vi "RT target - PWM Example.vi"() -> ()   [LabVIEW 2013]
uses:
  <vilib>/Platform/TimedLoop/XDataNode/timing_clust.ctl
  <vilib>/Platform/TimedLoop/XDataNode/nitl_modes.ctl
  <vilib>/Platform/TimedLoop/XDataNode/wakeup.ctl
  <vilib>/FPGAPlugInAG/cRIO-9068/niLvFpga_Open_cRIO-9068.vi
  <vilib>/Utility/error.llb/Error Cluster From Error Code.vi
  <vilib>/rvi/errors/niLvFpgaAdjustHostInterfaceError.vi
  <vilib>/FPGAPlugInAG/cRIO-9068/niLvFpga_Close_cRIO-9068.vi
  <vilib>/platform/TimedLoop/XDataNode/XDataNode.xnode
  <vilib>/rvi/interface/nirviOpenFPGA/nirviOpenFPGA.xnode
  FPGA Bitfiles/testscanmode_FPGATarget_FPGA-PWMExample_nwIUPoe6BIw.lvbitx
  FPGA - PWM Example.vi
  <vilib>/rvi/interface/nirviReadWriteControl/nirviReadWriteControl.xnode
  <vilib>/rvi/interface/nirviCloseFPGA/nirviCloseFPGA.xnode
  <vilib>/Platform/TimedLoop/XDataNode/XDNodeRunTimeDep.lvlib
  NiFpgaLv.dll
panel:
  in  "Array":bool[](array[boolean])
  out "error out":errorcluster
  in  "stop":bool
  # "Pulse Width Modulation (PWM)\nNI 9474 (Slot 4)"
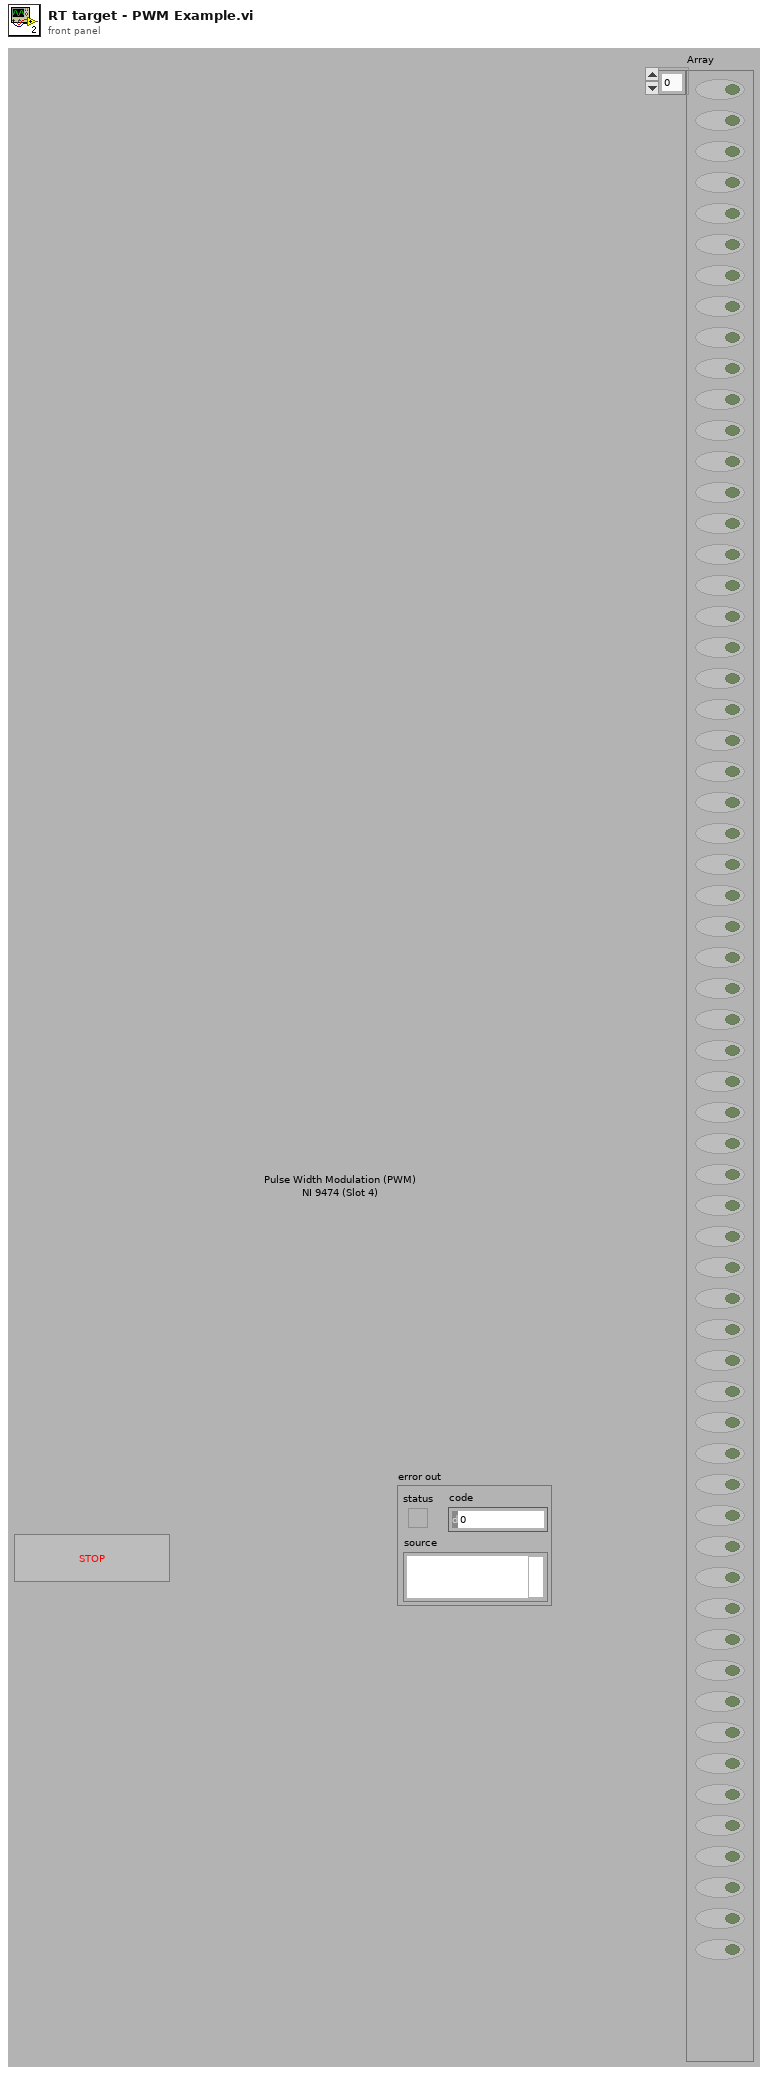
[diagram p1: front panel]
types:
  T1 = typedef "XDNodeRunTimeDep.lvlib/timing_clust.ctl" = cluster{"Expected End [f-1]":u64, "Actual End [f-1]":u64, "Finished Late? [f-1]":bool, "Expected End [i-1]":u64, "Actual End [i-1]":u64, "Finished Late? [i-1]":bool, "Expected Start [i]":u64, "Actual Start [i]":u64, "Expected Start [f]":u64, "Actual Start [f]":u64, "Source Name":string, "Structure Name":string, "Period":i64, "Deadline":i64, "Offset":i64, "Start":i64, "Priority":i32, "Timeout":i32, "Mode":T2, "Wakeup Reason":T3, "Error":errorcluster, "Source Type":string, "Secondary Source Type":string, "Global End Time":u64, "Global Start Time":u64, "Frame Duration":u64, "Iteration Duration":u64, "Assigned CPU":i32, "I/O Scan Engine Mode":u32}
  T2 = typedef "XDNodeRunTimeDep.lvlib/nitl_modes.ctl" = enum32{"No Change", "Process missed periods, maintain original phase", "Discard missed periods, maintain original phase", "Process missed periods, ignore original phase", "Discard missed periods, ignore original phase"}
  T3 = typedef "XDNodeRunTimeDep.lvlib/wakeup.ctl" = enum32{"Normal", "Aborted", "Asynchronous wakeup", "Timing source error", "Timed loop error", "Timeout"}
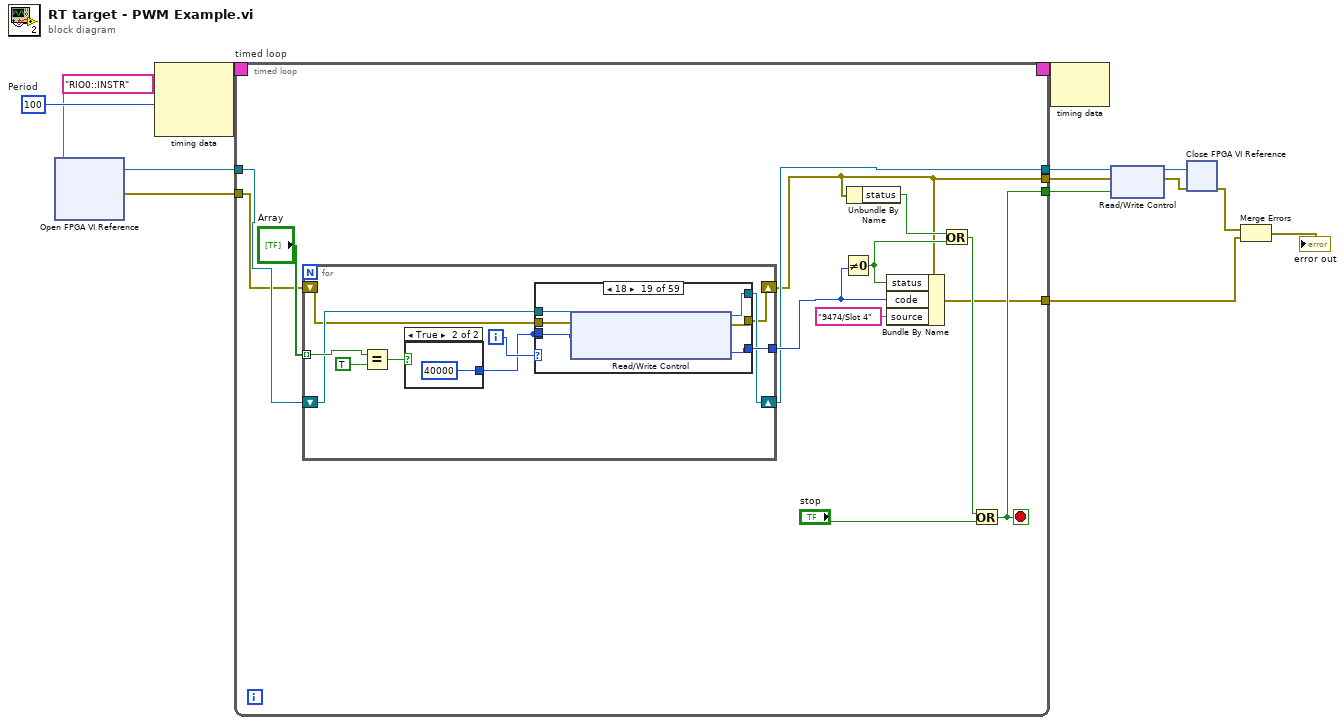
[diagram p0: block diagram]
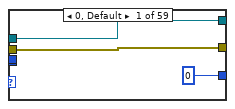
[diagram p2: hidden frame]
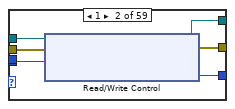
[diagram p3: hidden frame]
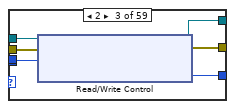
[diagram p4: hidden frame]
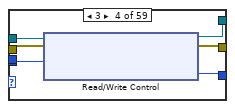
[diagram p5: hidden frame]
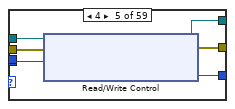
[diagram p6: hidden frame]
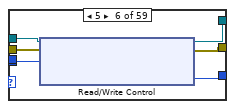
[diagram p7: hidden frame]
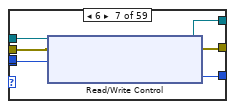
[diagram p8: hidden frame]
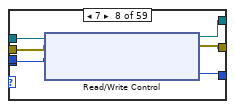
[diagram p9: hidden frame]
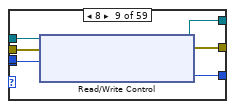
[diagram p10: hidden frame]
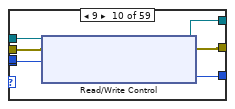
[diagram p11: hidden frame]
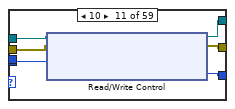
[diagram p12: hidden frame]
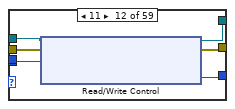
[diagram p13: hidden frame]
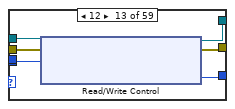
[diagram p14: hidden frame]
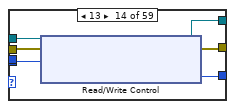
[diagram p15: hidden frame]
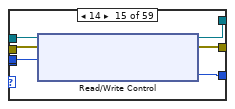
[diagram p16: hidden frame]
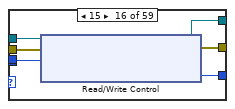
[diagram p17: hidden frame]
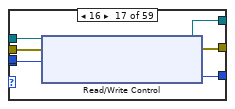
[diagram p18: hidden frame]
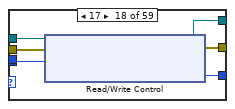
[diagram p19: hidden frame]
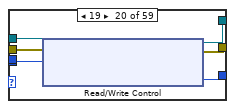
[diagram p20: hidden frame]
diagram:
  w12 = i64 100  # Period
  n1 = xnode "Open FPGA VI Reference"("resource name"=tag "RIO0::INSTR") -> ("FPGA VI Reference Out"=w11:refnum<k20>, "error out"=w10:errorcluster)  [unwired: 1 in]
  n2 = node-c288(w12) -> (w14:T1)  [unwired: 2 in]
  n3 = timed-loop "timed loop" {
    timing: w14 -> [_]
    timing-out: [_] -> w13
    tunnel: w11 -> [w19]
    tunnel: w10 -> [w18]
    tunnel: [w16] -> w1
    tunnel: [w15] -> w9
    tunnel: [w27] -> w6
    tunnel: [w21] -> w4
    stop <- w27 stop-if-true
    n4 = for {
      tunnel: "Array" -> [w35] mode=indexing
      tunnel: [w32] -> w17
      shift-right: [w30] -> w16
      shift-left: w19 -> [w33]
      shift-right: [w29] -> w15
      shift-left: w18 -> [w31]
      i -> [w34]
      n5 = Equal?(x=w35, y=TRUE) -> (x = y?=w37:bool)
      n6 = case shown="True" w37 {
        tunnel: [0 40000] -> w28
        frame False {
        }
        frame True {
        }
      }
      n7 = case shown="18" w34 {
        tunnel: w33 -> [w40 w46 w49 w53 w64 w70 w76 w82 w85 w91 w100 w106 w112 w118 w124 w130 w136 w142 w148 w154 w160 w166 w172 w178 w184 w190 w196 w202 w208 w214 w220 w226 w232 w238 w244 w250 w251 w262 w268 w274 w280 w286 w292 w298 w304 w310 w316 w322 w328 w334 w340 w346 w352 w358 w364 w370 w376 w382 w388]
        tunnel: [0 ("9401/Slot 3 Error Code") w45 w50 w55 w59 w65 w71 w79 w86 w92 w95 w101 w107 w113 w119 w125 w131 w137 w144 w149 w155 w161 w167 w173 w179 w185 w191 w197 w203 w209 w215 w221 w227 w233 w239 w245 w252 w257 w263 w269 w275 w281 w287 w293 w299 w305 w311 w317 w323 w329 w335 w341 w347 w353 w359 w365 w371 w377 w383] -> w32
        tunnel: [w40 w43 w52 w57 w61 w67 w73 w77 w88 w94 w97 w103 w109 w115 w121 w127 w133 w139 w143 w151 w157 w163 w169 w175 w181 w187 w193 w199 w205 w211 w217 w223 w229 w235 w241 w247 w254 w259 w265 w271 w277 w283 w289 w295 w301 w307 w313 w319 w325 w331 w337 w343 w349 w355 w361 w367 w373 w379 w385] -> w30
        tunnel: w31 -> [w38 w44 w48 w58 w63 w69 w75 w81 w84 w90 w99 w105 w111 w117 w123 w129 w135 w141 w147 w153 w159 w165 w171 w177 w183 w189 w195 w201 w207 w213 w219 w225 w231 w237 w243 w249 w256 w261 w267 w273 w279 w285 w291 w297 w303 w309 w315 w321 w327 w333 w339 w345 w351 w357 w363 w369 w375 w381 w387]
        tunnel: [w38 w42 w51 w56 w60 w66 w72 w78 w87 w93 w96 w102 w108 w114 w120 w126 w132 w138 w145 w150 w156 w162 w168 w174 w180 w186 w192 w198 w204 w210 w216 w222 w228 w234 w240 w246 w253 w258 w264 w270 w276 w282 w288 w294 w300 w306 w312 w318 w324 w330 w336 w342 w348 w354 w360 w366 w372 w378 w384] -> w29
        tunnel: w28 -> [_ w41 w47 w54 w62 w68 w74 w80 w83 w89 w98 w104 w110 w116 _ w128 w134 w140 w146 w152 w158 w164 w170 w176 w182 w188 w194 w200 w206 w212 w218 w224 w230 w236 w242 w248 w255 w260 w266 w272 w278 w284 w290 w296 w302 w308 w314 w320 w326 w332 w338 w344 w350 w356 w362 w368 w374 w380 w386]
        tunnel: w28 -> [_ _ _ _ _ _ _ _ _ _ _ _ _ _ w122 _ _ _ _ _ _ _ _ _ _ _ _ _ _ _ _ _ _ _ _ _ _ _ _ _ _ _ _ _ _ _ _ _ _ _ _ _ _ _ _ _ _ _ _]
        frame 0, Default {
        }
        frame 1 {
          n8 = xnode "Read/Write Control"("FPGA VI Reference In"=w46, "error in"=w44, "PWM Duty Cycle (Ticks) 1"=w41) -> ("FPGA VI Reference Out"=w43:refnum<k20>, "error out"=w42:errorcluster, "9401/Slot 3 Error Code"=w45:i32)
        }
        frame 2 {
          n9 = xnode "Read/Write Control"("FPGA VI Reference In"=w49, "error in"=w48, "PWM Duty Cycle (Ticks) 2"=w47) -> ("FPGA VI Reference Out"=w52:refnum<k20>, "error out"=w51:errorcluster, "9401/Slot 3 Error Code"=w50:i32)
        }
        frame 3 {
          n10 = xnode "Read/Write Control"("FPGA VI Reference In"=w53, "error in"=w58, "PWM Duty Cycle (Ticks) 3"=w54) -> ("FPGA VI Reference Out"=w57:refnum<k20>, "error out"=w56:errorcluster, "9401/Slot 3 Error Code"=w55:i32)
        }
        frame 4 {
          n11 = xnode "Read/Write Control"("FPGA VI Reference In"=w64, "error in"=w63, "PWM Duty Cycle (Ticks) 4"=w62) -> ("FPGA VI Reference Out"=w61:refnum<k20>, "error out"=w60:errorcluster, "9401/Slot 3 Error Code"=w59:i32)
        }
        frame 5 {
          n12 = xnode "Read/Write Control"("FPGA VI Reference In"=w70, "error in"=w69, "PWM Duty Cycle (Ticks) 5"=w68) -> ("FPGA VI Reference Out"=w67:refnum<k20>, "error out"=w66:errorcluster, "9401/Slot 3 Error Code"=w65:i32)
        }
        frame 6 {
          n13 = xnode "Read/Write Control"("FPGA VI Reference In"=w76, "error in"=w75, "PWM Duty Cycle (Ticks) 6"=w74) -> ("FPGA VI Reference Out"=w73:refnum<k20>, "error out"=w72:errorcluster, "9401/Slot 3 Error Code"=w71:i32)
        }
        frame 7 {
          n14 = xnode "Read/Write Control"("FPGA VI Reference In"=w82, "error in"=w81, "PWM Duty Cycle (Ticks) 7"=w80) -> ("FPGA VI Reference Out"=w77:refnum<k20>, "error out"=w78:errorcluster, "9401/Slot 3 Error Code"=w79:i32)
        }
        frame 8 {
          n15 = xnode "Read/Write Control"("FPGA VI Reference In"=w85, "error in"=w84, "PWM Duty Cycle (Ticks) 8"=w83) -> ("FPGA VI Reference Out"=w88:refnum<k20>, "error out"=w87:errorcluster, "9401/Slot 3 Error Code"=w86:i32)
        }
        frame 9 {
          n16 = xnode "Read/Write Control"("FPGA VI Reference In"=w91, "error in"=w90, "PWM Duty Cycle (Ticks) 9"=w89) -> ("FPGA VI Reference Out"=w94:refnum<k20>, "error out"=w93:errorcluster, "9401/Slot 3 Error Code"=w92:i32)
        }
        frame 10 {
          n17 = xnode "Read/Write Control"("FPGA VI Reference In"=w100, "error in"=w99, "PWM Duty Cycle (Ticks) 10"=w98) -> ("FPGA VI Reference Out"=w97:refnum<k20>, "error out"=w96:errorcluster, "9401/Slot 3 Error Code"=w95:i32)
        }
        frame 11 {
          n18 = xnode "Read/Write Control"("FPGA VI Reference In"=w106, "error in"=w105, "PWM Duty Cycle (Ticks) 11"=w104) -> ("FPGA VI Reference Out"=w103:refnum<k20>, "error out"=w102:errorcluster, "9401/Slot 3 Error Code"=w101:i32)
        }
        frame 12 {
          n19 = xnode "Read/Write Control"("FPGA VI Reference In"=w112, "error in"=w111, "PWM Duty Cycle (Ticks) 12"=w110) -> ("FPGA VI Reference Out"=w109:refnum<k20>, "error out"=w108:errorcluster, "9401/Slot 3 Error Code"=w107:i32)
        }
        frame 13 {
          n20 = xnode "Read/Write Control"("FPGA VI Reference In"=w118, "error in"=w117, "PWM Duty Cycle (Ticks) 13"=w116) -> ("FPGA VI Reference Out"=w115:refnum<k20>, "error out"=w114:errorcluster, "9401/Slot 3 Error Code"=w113:i32)
        }
        frame 14 {
          n21 = xnode "Read/Write Control"("FPGA VI Reference In"=w124, "error in"=w123, "PWM Duty Cycle (Ticks) 14"=w122) -> ("FPGA VI Reference Out"=w121:refnum<k20>, "error out"=w120:errorcluster, "9401/Slot 3 Error Code"=w119:i32)
        }
        frame 15 {
          n22 = xnode "Read/Write Control"("FPGA VI Reference In"=w130, "error in"=w129, "PWM Duty Cycle (Ticks) 15"=w128) -> ("FPGA VI Reference Out"=w127:refnum<k20>, "error out"=w126:errorcluster, "9401/Slot 3 Error Code"=w125:i32)
        }
        frame 16 {
          n23 = xnode "Read/Write Control"("FPGA VI Reference In"=w136, "error in"=w135, "PWM Duty Cycle (Ticks) 16"=w134) -> ("FPGA VI Reference Out"=w133:refnum<k20>, "error out"=w132:errorcluster, "9401/Slot 3 Error Code"=w131:i32)
        }
        frame 17 {
          n24 = xnode "Read/Write Control"("FPGA VI Reference In"=w142, "error in"=w141, "PWM Duty Cycle (Ticks) 17"=w140) -> ("FPGA VI Reference Out"=w139:refnum<k20>, "error out"=w138:errorcluster, "9401/Slot 3 Error Code"=w137:i32)
        }
        frame 18 {
          n25 = xnode "Read/Write Control"("FPGA VI Reference In"=w148, "error in"=w147, "PWM Duty Cycle (Ticks) 18"=w146) -> ("FPGA VI Reference Out"=w143:refnum<k20>, "error out"=w145:errorcluster, "9401/Slot 3 Error Code"=w144:i32)
        }
        frame 19 {
          n26 = xnode "Read/Write Control"("FPGA VI Reference In"=w154, "error in"=w153, "PWM Duty Cycle (Ticks) 19"=w152) -> ("FPGA VI Reference Out"=w151:refnum<k20>, "error out"=w150:errorcluster, "9401/Slot 3 Error Code"=w149:i32)
        }
        frame 20 {
          n27 = xnode "Read/Write Control"("FPGA VI Reference In"=w160, "error in"=w159, "PWM Duty Cycle (Ticks) 20"=w158) -> ("FPGA VI Reference Out"=w157:refnum<k20>, "error out"=w156:errorcluster, "9401/Slot 3 Error Code"=w155:i32)
        }
        frame 21 {
          n28 = xnode "Read/Write Control"("FPGA VI Reference In"=w166, "error in"=w165, "PWM Duty Cycle (Ticks) 21"=w164) -> ("FPGA VI Reference Out"=w163:refnum<k20>, "error out"=w162:errorcluster, "9401/Slot 3 Error Code"=w161:i32)
        }
        frame 22 {
          n29 = xnode "Read/Write Control"("FPGA VI Reference In"=w172, "error in"=w171, "PWM Duty Cycle (Ticks) 22"=w170) -> ("FPGA VI Reference Out"=w169:refnum<k20>, "error out"=w168:errorcluster, "9401/Slot 3 Error Code"=w167:i32)
        }
        frame 23 {
          n30 = xnode "Read/Write Control"("FPGA VI Reference In"=w178, "error in"=w177, "PWM Duty Cycle (Ticks) 23"=w176) -> ("FPGA VI Reference Out"=w175:refnum<k20>, "error out"=w174:errorcluster, "9401/Slot 3 Error Code"=w173:i32)
        }
        frame 24 {
          n31 = xnode "Read/Write Control"("FPGA VI Reference In"=w184, "error in"=w183, "PWM Duty Cycle (Ticks) 24"=w182) -> ("FPGA VI Reference Out"=w181:refnum<k20>, "error out"=w180:errorcluster, "9401/Slot 3 Error Code"=w179:i32)
        }
        frame 25 {
          n32 = xnode "Read/Write Control"("FPGA VI Reference In"=w190, "error in"=w189, "PWM Duty Cycle (Ticks) 25"=w188) -> ("FPGA VI Reference Out"=w187:refnum<k20>, "error out"=w186:errorcluster, "9401/Slot 3 Error Code"=w185:i32)
        }
        frame 26 {
          n33 = xnode "Read/Write Control"("FPGA VI Reference In"=w196, "error in"=w195, "PWM Duty Cycle (Ticks) 26"=w194) -> ("FPGA VI Reference Out"=w193:refnum<k20>, "error out"=w192:errorcluster, "9401/Slot 3 Error Code"=w191:i32)
        }
        frame 27 {
          n34 = xnode "Read/Write Control"("FPGA VI Reference In"=w202, "error in"=w201, "PWM Duty Cycle (Ticks) 27"=w200) -> ("FPGA VI Reference Out"=w199:refnum<k20>, "error out"=w198:errorcluster, "9401/Slot 3 Error Code"=w197:i32)
        }
        frame 28 {
          n35 = xnode "Read/Write Control"("FPGA VI Reference In"=w208, "error in"=w207, "PWM Duty Cycle (Ticks) 28"=w206) -> ("FPGA VI Reference Out"=w205:refnum<k20>, "error out"=w204:errorcluster, "9401/Slot 3 Error Code"=w203:i32)
        }
        frame 29 {
          n36 = xnode "Read/Write Control"("FPGA VI Reference In"=w214, "error in"=w213, "PWM Duty Cycle (Ticks) 29"=w212) -> ("FPGA VI Reference Out"=w211:refnum<k20>, "error out"=w210:errorcluster, "9401/Slot 3 Error Code"=w209:i32)
        }
        frame 30 {
          n37 = xnode "Read/Write Control"("FPGA VI Reference In"=w220, "error in"=w219, "PWM Duty Cycle (Ticks) 30"=w218) -> ("FPGA VI Reference Out"=w217:refnum<k20>, "error out"=w216:errorcluster, "9401/Slot 3 Error Code"=w215:i32)
        }
        frame 31 {
          n38 = xnode "Read/Write Control"("FPGA VI Reference In"=w226, "error in"=w225, "PWM Duty Cycle (Ticks) 31"=w224) -> ("FPGA VI Reference Out"=w223:refnum<k20>, "error out"=w222:errorcluster, "9401/Slot 3 Error Code"=w221:i32)
        }
        frame 32 {
          n39 = xnode "Read/Write Control"("FPGA VI Reference In"=w232, "error in"=w231, "PWM Duty Cycle (Ticks) 32"=w230) -> ("FPGA VI Reference Out"=w229:refnum<k20>, "error out"=w228:errorcluster, "9401/Slot 3 Error Code"=w227:i32)
        }
        frame 33 {
          n40 = xnode "Read/Write Control"("FPGA VI Reference In"=w238, "error in"=w237, "PWM Duty Cycle (Ticks) 33"=w236) -> ("FPGA VI Reference Out"=w235:refnum<k20>, "error out"=w234:errorcluster, "9401/Slot 3 Error Code"=w233:i32)
        }
        frame 34 {
          n41 = xnode "Read/Write Control"("FPGA VI Reference In"=w244, "error in"=w243, "PWM Duty Cycle (Ticks) 34"=w242) -> ("FPGA VI Reference Out"=w241:refnum<k20>, "error out"=w240:errorcluster, "9401/Slot 3 Error Code"=w239:i32)
        }
        frame 35 {
          n42 = xnode "Read/Write Control"("FPGA VI Reference In"=w250, "error in"=w249, "PWM Duty Cycle (Ticks) 35"=w248) -> ("FPGA VI Reference Out"=w247:refnum<k20>, "error out"=w246:errorcluster, "9401/Slot 3 Error Code"=w245:i32)
        }
        frame 36 {
          n43 = xnode "Read/Write Control"("FPGA VI Reference In"=w251, "error in"=w256, "PWM Duty Cycle (Ticks) 36"=w255) -> ("FPGA VI Reference Out"=w254:refnum<k20>, "error out"=w253:errorcluster, "9401/Slot 3 Error Code"=w252:i32)
        }
        frame 37 {
          n44 = xnode "Read/Write Control"("FPGA VI Reference In"=w262, "error in"=w261, "PWM Duty Cycle (Ticks) 37"=w260) -> ("FPGA VI Reference Out"=w259:refnum<k20>, "error out"=w258:errorcluster, "9401/Slot 3 Error Code"=w257:i32)
        }
        frame 38 {
          n45 = xnode "Read/Write Control"("FPGA VI Reference In"=w268, "error in"=w267, "PWM Duty Cycle (Ticks) 38"=w266) -> ("FPGA VI Reference Out"=w265:refnum<k20>, "error out"=w264:errorcluster, "9401/Slot 3 Error Code"=w263:i32)
        }
        frame 39 {
          n46 = xnode "Read/Write Control"("FPGA VI Reference In"=w274, "error in"=w273, "PWM Duty Cycle (Ticks) 39"=w272) -> ("FPGA VI Reference Out"=w271:refnum<k20>, "error out"=w270:errorcluster, "9401/Slot 3 Error Code"=w269:i32)
        }
        frame 40 {
          n47 = xnode "Read/Write Control"("FPGA VI Reference In"=w280, "error in"=w279, "PWM Duty Cycle (Ticks) 40"=w278) -> ("FPGA VI Reference Out"=w277:refnum<k20>, "error out"=w276:errorcluster, "9401/Slot 3 Error Code"=w275:i32)
        }
        frame 41 {
          n48 = xnode "Read/Write Control"("FPGA VI Reference In"=w286, "error in"=w285, "PWM Duty Cycle (Ticks) 41"=w284) -> ("FPGA VI Reference Out"=w283:refnum<k20>, "error out"=w282:errorcluster, "9401/Slot 3 Error Code"=w281:i32)
        }
        frame 42 {
          n49 = xnode "Read/Write Control"("FPGA VI Reference In"=w292, "error in"=w291, "PWM Duty Cycle (Ticks) 42"=w290) -> ("FPGA VI Reference Out"=w289:refnum<k20>, "error out"=w288:errorcluster, "9401/Slot 3 Error Code"=w287:i32)
        }
        frame 43 {
          n50 = xnode "Read/Write Control"("FPGA VI Reference In"=w298, "error in"=w297, "PWM Duty Cycle (Ticks) 43"=w296) -> ("FPGA VI Reference Out"=w295:refnum<k20>, "error out"=w294:errorcluster, "9401/Slot 3 Error Code"=w293:i32)
        }
        frame 44 {
          n51 = xnode "Read/Write Control"("FPGA VI Reference In"=w304, "error in"=w303, "PWM Duty Cycle (Ticks) 44"=w302) -> ("FPGA VI Reference Out"=w301:refnum<k20>, "error out"=w300:errorcluster, "9401/Slot 3 Error Code"=w299:i32)
        }
        frame 45 {
          n52 = xnode "Read/Write Control"("FPGA VI Reference In"=w310, "error in"=w309, "PWM Duty Cycle (Ticks) 45"=w308) -> ("FPGA VI Reference Out"=w307:refnum<k20>, "error out"=w306:errorcluster, "9401/Slot 3 Error Code"=w305:i32)
        }
        frame 46 {
          n53 = xnode "Read/Write Control"("FPGA VI Reference In"=w316, "error in"=w315, "PWM Duty Cycle (Ticks) 46"=w314) -> ("FPGA VI Reference Out"=w313:refnum<k20>, "error out"=w312:errorcluster, "9401/Slot 3 Error Code"=w311:i32)
        }
        frame 47 {
          n54 = xnode "Read/Write Control"("FPGA VI Reference In"=w322, "error in"=w321, "PWM Duty Cycle (Ticks) 47"=w320) -> ("FPGA VI Reference Out"=w319:refnum<k20>, "error out"=w318:errorcluster, "9401/Slot 3 Error Code"=w317:i32)
        }
        frame 48 {
          n55 = xnode "Read/Write Control"("FPGA VI Reference In"=w328, "error in"=w327, "PWM Duty Cycle (Ticks) 48"=w326) -> ("FPGA VI Reference Out"=w325:refnum<k20>, "error out"=w324:errorcluster, "9401/Slot 3 Error Code"=w323:i32)
        }
        frame 49 {
          n56 = xnode "Read/Write Control"("FPGA VI Reference In"=w334, "error in"=w333, "PWM Duty Cycle (Ticks) 49"=w332) -> ("FPGA VI Reference Out"=w331:refnum<k20>, "error out"=w330:errorcluster, "9401/Slot 3 Error Code"=w329:i32)
        }
        frame 50 {
          n57 = xnode "Read/Write Control"("FPGA VI Reference In"=w340, "error in"=w339, "PWM Duty Cycle (Ticks) 50"=w338) -> ("FPGA VI Reference Out"=w337:refnum<k20>, "error out"=w336:errorcluster, "9401/Slot 3 Error Code"=w335:i32)
        }
        frame 51 {
          n58 = xnode "Read/Write Control"("FPGA VI Reference In"=w346, "error in"=w345, "PWM Duty Cycle (Ticks) 51"=w344) -> ("FPGA VI Reference Out"=w343:refnum<k20>, "error out"=w342:errorcluster, "9401/Slot 3 Error Code"=w341:i32)
        }
        frame 52 {
          n59 = xnode "Read/Write Control"("FPGA VI Reference In"=w352, "error in"=w351, "PWM Duty Cycle (Ticks) 52"=w350) -> ("FPGA VI Reference Out"=w349:refnum<k20>, "error out"=w348:errorcluster, "9401/Slot 3 Error Code"=w347:i32)
        }
        frame 53 {
          n60 = xnode "Read/Write Control"("FPGA VI Reference In"=w358, "error in"=w357, "PWM Duty Cycle (Ticks) 53"=w356) -> ("FPGA VI Reference Out"=w355:refnum<k20>, "error out"=w354:errorcluster, "9401/Slot 3 Error Code"=w353:i32)
        }
        frame 54 {
          n61 = xnode "Read/Write Control"("FPGA VI Reference In"=w364, "error in"=w363, "PWM Duty Cycle (Ticks) 54"=w362) -> ("FPGA VI Reference Out"=w361:refnum<k20>, "error out"=w360:errorcluster, "9401/Slot 3 Error Code"=w359:i32)
        }
        frame 55 {
          n62 = xnode "Read/Write Control"("FPGA VI Reference In"=w370, "error in"=w369, "PWM Duty Cycle (Ticks) 55"=w368) -> ("FPGA VI Reference Out"=w367:refnum<k20>, "error out"=w366:errorcluster, "9401/Slot 3 Error Code"=w365:i32)
        }
        frame 56 {
          n63 = xnode "Read/Write Control"("FPGA VI Reference In"=w376, "error in"=w375, "PWM Duty Cycle (Ticks) 56"=w374) -> ("FPGA VI Reference Out"=w373:refnum<k20>, "error out"=w372:errorcluster, "9401/Slot 3 Error Code"=w371:i32)
        }
        frame 57 {
          n64 = xnode "Read/Write Control"("FPGA VI Reference In"=w382, "error in"=w381, "PWM Duty Cycle (Ticks) 57"=w380) -> ("FPGA VI Reference Out"=w379:refnum<k20>, "error out"=w378:errorcluster, "9401/Slot 3 Error Code"=w377:i32)
        }
        frame 58 {
          n65 = xnode "Read/Write Control"("FPGA VI Reference In"=w388, "error in"=w387, "PWM Duty Cycle (Ticks) 58"=w386) -> ("FPGA VI Reference Out"=w385:refnum<k20>, "error out"=w384:errorcluster, "9401/Slot 3 Error Code"=w383:i32)
        }
      }
    }
    n66 = Not Equal To 0?(x=w17) -> (x != 0?=w23:bool)
    n67 = Unbundle By Name(w15) -> ("status"=w25:bool)
    n68 = Bundle By Name(cluster=w15, "status"=w23, "code"=w17, "source"="9474/Slot 4") -> (w21:errorcluster)
    n69 = Or(x=w25, y=w23) -> (x .or. y?=w24:bool)
    n70 = Or(x=w24, y="stop") -> (x .or. y?=w27:bool)
  }
  n71 = node-c288(w13) -> ()  [unwired: 1 out]
  n72 = xnode "Read/Write Control"("FPGA VI Reference In"=w1, "error in"=w9, "stop"=w6) -> ("FPGA VI Reference Out"=w8:refnum<k20>, "error out"=w7:errorcluster)
  n73 = xnode "Close FPGA VI Reference"("FPGA VI Reference In"=w8, "error in"=w7) -> ("error out"=w5:errorcluster)
  n74 = Merge Errors(w5, w4) -> (→"error out":errorcluster)
